vi "TDT-Set Target Val.vi"   [LabVIEW 2015]
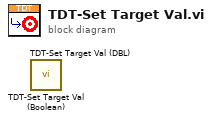
[diagram p0: block diagram]
diagram:
  n1 = call "TDT-Set Target Val (Boolean).vi"() -> ()  [unwired: 15 in, 1 out]
  n2 = call "TDT-Set Target Val (DBL).vi"() -> ()  [unwired: 15 in, 1 out]
